vi "Pack For Grpc.vi"(8 "error in (no error)":errorcluster, 9 "Configuration / Resuls (Config)":enum16{"Configuration", "Results"}(ring), 10 "Data Value":variant, 11 "MeasurementPluginService in":refnum<class "Fake Measurement Plugin.lvclass">) -> (0 "error out":errorcluster, 2 "Any":T1, 3 "MeasurementPluginService out":refnum<class "Fake Measurement Plugin.lvclass">)   [LabVIEW 2020, in "MeasurementServerTests.lvlib" / "Measurement Plugin Service Tests.lvlib" / "Fake Measurement Plugin.lvclass"]
uses:
  Fake Measurement Plugin.lvclass
  <vilib>/gRPC/LabVIEW gRPC Library/Shared/Any.ctl
  Runtime/MeasurementLink Measurement Server/Measurement Plugin Service/Measurement Plugin Service.lvclass
  <vilib>/gRPC/LabVIEW gRPC Library/grpc-lvsupport-release.lvlib
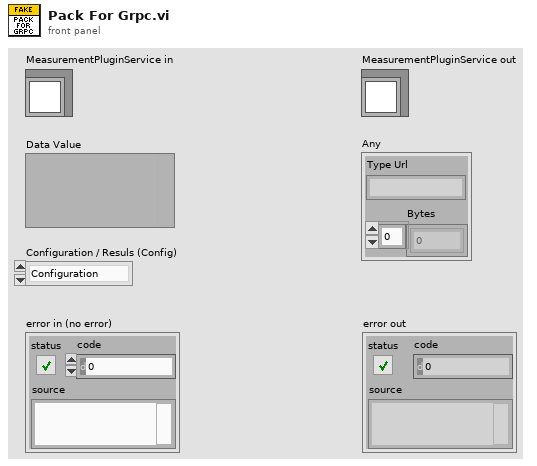
[diagram p1: front panel]
types:
  T1 = typedef "grpc-lvsupport-release.lvlib/Any.ctl" = cluster{"Type Url":string, "Bytes":u8[]}
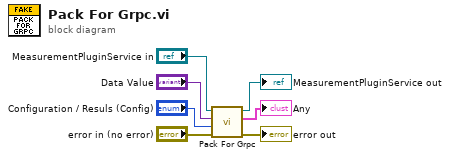
[diagram p0: block diagram]
diagram:
  n1 = call-parent "Pack For Grpc.vi"("error in (no error)"="error in (no error)", "Configuration / Resuls (Config)"="Configuration / Resuls (Config)", "Data Value"="Data Value", "MeasurementPluginService in"="MeasurementPluginService in") -> ("error out"=→"error out":errorcluster, "Any"=→"Any":T1, "MeasurementPluginService out"=→"MeasurementPluginService out":refnum<class "Fake Measurement Plugin.lvclass">)  [unwired: 5 in]
